vi "OE1022D_OpenDevice.vi"(0 "VISA resource name":refnum<visa-resource-name>) -> (14 "VISA资源名称输出":refnum<visa-resource-name>, 19 "错误输出":errorcluster)   [LabVIEW 2022 SP3]
doc: "Configures the reference source and the internal oscillator."
uses:
  <vilib>/Instr/_visa.llb/VISA Configure Serial Port (Instr).vi
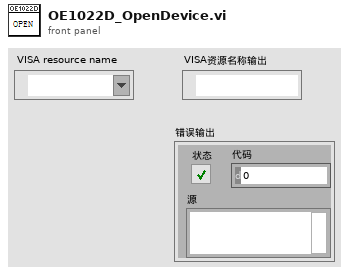
[diagram p1: front panel]
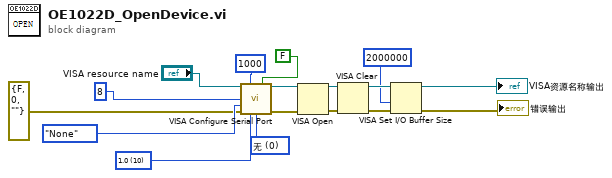
[diagram p0: block diagram]
diagram:
  w5 = u16 0 items=["无", "XON/XOFF", "RTS/CTS", "XON/XOFF & RTS/CTS", "DTR/DSR", "XON/XOFF & DTR/DSR"] ("flow control (0:none)")
  w6 = u16 10 items=["1.0"=10, "1.5"=15, "2.0"=20] ("stop bits (10: 1 bit)")
  n1 = call-poly "VISA Configure Serial Port"("VISA resource name"="VISA resource name", "timeout (10sec)"=u32 1000, "Enable Termination\nChar (T)"=FALSE ("Enable Termination\nChar (T)"), "data bits (8)"=u16 8, "parity (0:none)"=enum16{"None", "Odd", "Even", "Mark", "Space"}."None", "error in (no error)"=errorcluster {"status"=FALSE, "code"=0, "source"=""} ("error out"), "stop bits (10: 1 bit)"=w6, "flow control (0:none)"=w5) -> ("VISA resource name out"=w15:refnum<visa-resource-name>, "error out"=w14:errorcluster)  [unwired: 6 in]
  n2 = VISA Open(error in (no error)=w14, VISA resource name=w15) -> (VISA resource name=w16:refnum<visa-resource-name>, error out=w17:errorcluster)  [unwired: 3 in]
  n3 = VISA Clear(VISA resource name=w16, error in (no error)=w17) -> (VISA resource name out=w12:refnum<visa-resource-name>, error out=w13:errorcluster)
  n4 = VISA Set I/O Buffer Size(VISA resource name=w12, size (4096)=u32 2000000 ("大小(4096)"), error in (no error)=w13) -> (VISA resource name out=→"VISA资源名称输出":refnum<visa-resource-name>, error out=→"错误输出":errorcluster)  [unwired: 1 in]
